vi "FindParetheses.vi"(0 "String in":string) -> (1 "rest":string, 2 "parentetical":string)   [LabVIEW 2014]
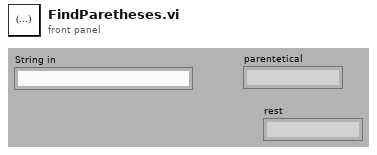
[diagram p1: front panel]
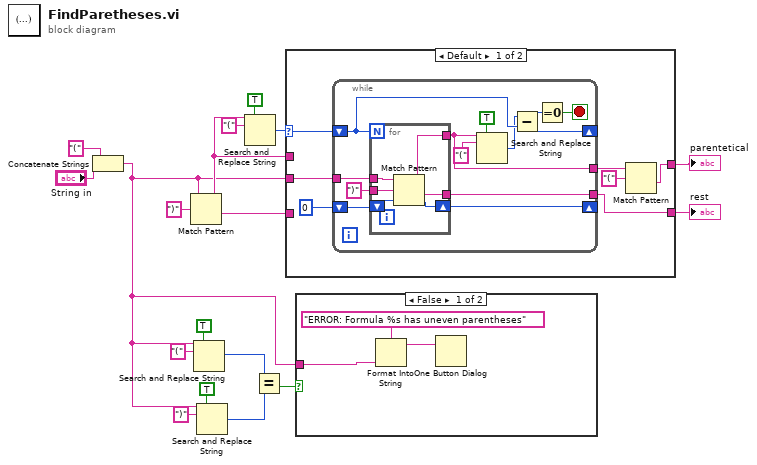
[diagram p0: block diagram]
diagram:
  n1 = Concatenate Strings("(" ("string"), "String in") -> (w4:string)
  n2 = Match Pattern(string=w4, regular expression=")") -> (before substring=w14:string, after substring=w13:string)  [unwired: 1 in, 2 out]
  n3 = Search and Replace String(replace all?=TRUE ("replace all? (F)"), input string=w4, search string="(" ("regular expression")) -> (number of replacements=w2:i32)  [unwired: 5 in, 3 out]
  n4 = Search and Replace String(replace all?=TRUE ("replace all? (F)"), input string=w4, search string=")" ("regular expression")) -> (number of replacements=w7:i32)  [unwired: 5 in, 3 out]
  n5 = Search and Replace String(replace all?=TRUE ("replace all? (F)"), input string=w14, search string="(" ("regular expression")) -> (number of replacements=w16:i32)  [unwired: 5 in, 3 out]
  n6 = Equal?(x=w2, y=w7) -> (x = y?=w6:bool)
  n7 = case shown="Default" w16 {
    selector: w16 -> [w23 _]
    tunnel: [w19 w45] -> w15
    tunnel: w14 -> [_ w45]
    tunnel: w13 -> [_ w44]
    tunnel: w4 -> [w24 _]
    tunnel: [w22 w44] -> w1
    frame Default {
      n8 = while {
        tunnel: w24 -> [w35]
        shift-right: [w34] -> _
        shift-left: 0 ("offset past match") -> [w36]
        shift-right: [w30] -> _
        shift-left: w23 -> [w29]
        tunnel: [w27] -> w22
        tunnel: [w26] -> w20
        stop <- w31 stop-if-true
        n9 = for {
          N: w29 -> [_]
          tunnel: w35 -> [w43]
          tunnel: ")" ("regular expression") -> [w42]
          shift-right: [w41] -> w34
          shift-left: w36 -> [w40]
          tunnel: [w39] -> w26
          tunnel: [w38] -> w27
          n10 = Match Pattern(string=w43, regular expression=w42, offset (0)=w40) -> (before substring=w39:string, after substring=w38:string, offset past match=w41:i32)  [unwired: 1 out]
        }
        n11 = Search and Replace String(replace all?=TRUE ("replace all? (F)"), input string=w26, search string="(" ("regular expression")) -> (number of replacements=w28:i32)  [unwired: 5 in, 3 out]
        n12 = Subtract(x=w28, y=w29) -> (x-y=w30:i32)
        n13 = Equal To 0?(x=w30) -> (x = 0?=w31:bool)
      }
      n14 = Match Pattern(string=w20, regular expression="(") -> (after substring=w19:string)  [unwired: 1 in, 3 out]
    }
    frame 0 {
    }
  }
  "parentetical" <- w15
  "rest" <- w1
  n15 = case shown="False" w6 {
    tunnel: w4 -> [w47 _]
    frame False {
      n16 = Format Into String(format string="ERROR: Formula %s has uneven parentheses", w47) -> (resulting string=w46:string)  [unwired: 2 in, 1 out]
      n17 = One Button Dialog(message=w46) -> ()  [unwired: 1 in, 1 out]
    }
    frame True {
    }
  }
